vi "stop acquisition.vi"(8 "error in (no error)":errorcluster, 11 "IMAQdx Cam in":refnum<class "IMAQdx Cam.lvclass">) -> (0 "error out":errorcluster, 3 "IMAQdx Cam out":refnum<class "IMAQdx Cam.lvclass">)   [LabVIEW 2020, in "IMAQdx Cam.lvclass"]
uses:
  IMAQdx Cam.lvclass
  IMAQdx Cam.lvclass/IMAQdx Cam.ctl
  <vilib>/vision/driver/NI_Vision_Acquisition_Software.lvlib
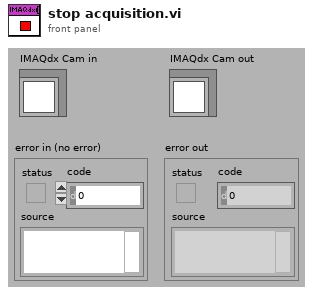
[diagram p1: front panel]
types:
  T1 = typedef "IMAQdx.ctl" = refnum<k21>
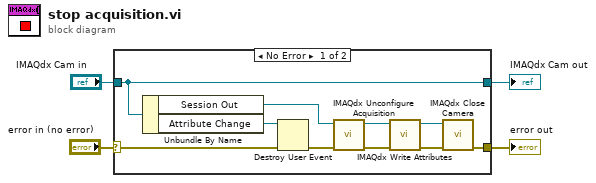
[diagram p0: block diagram]
diagram:
  n1 = case shown="No Error" "error in (no error)" {
    selector: "error in (no error)" -> [w11 w16]
    tunnel: [w13 w16] -> w3
    tunnel: [w14 w15] -> w1
    tunnel: "IMAQdx Cam in" -> [w14 w15]
    frame No Error {
      n2 = Unbundle By Name(w14) -> ("Session Out"=w10:T1, "Attribute Change"=w12:refnum<user-event>)
      n3 = Destroy User Event(user event=w12, error in=w11) -> (error out=w9:errorcluster)
      n4 = call <vilib>:"IMAQdx Unconfigure Acquisition.vi"("error in"=w9, "Session In"=w10) -> ("error out"=w7:errorcluster, "Session Out"=w8:T1)  [unwired: 8 out]
      n5 = call <vilib>:"IMAQdx Write Attributes.vi"("error in"=w7, "Session In"=w8) -> ("error out"=w6:errorcluster, "Session Out"=w5:T1)  [unwired: 8 in]
      n6 = call <vilib>:"IMAQdx Close Camera.vi"("error in"=w6, "Session In"=w5) -> ("error out"=w13:errorcluster)  [unwired: 9 out]
    }
    frame Error {
    }
  }
  "error out" <- w3
  "IMAQdx Cam out" <- w1
